vi "Normalized Axes.vi"(8 "axis in":T3, 11 "Device in":T1={"device ID"=refnum, "Device Name"="Logitech Extreme 3D", "axis info"={"X axis"=[], "Y axis"=[], "Z axis"=[], "X axis rotation"=[], "Y axis rotation"=[], "Z axis rotation"=[], "U axis"=[], "V axis"=[]}}) -> (0 "axis out":T2, 3 "Device out":T1={"device ID"=refnum, "Device Name"="Logitech Extreme 3D", "axis info"={"X axis"=[], "Y axis"=[], "Z axis"=[], "X axis rotation"=[], "Y axis rotation"=[], "Z axis rotation"=[], "U axis"=[], "V axis"=[]}})   [LabVIEW 2012]
doc: "This VI is used to normalize the newly reed axis info utilizing past minimums and maximums found during the calibration process. This ensures that the control input remains within the bounded range of 1 to -1.\nRuffin"
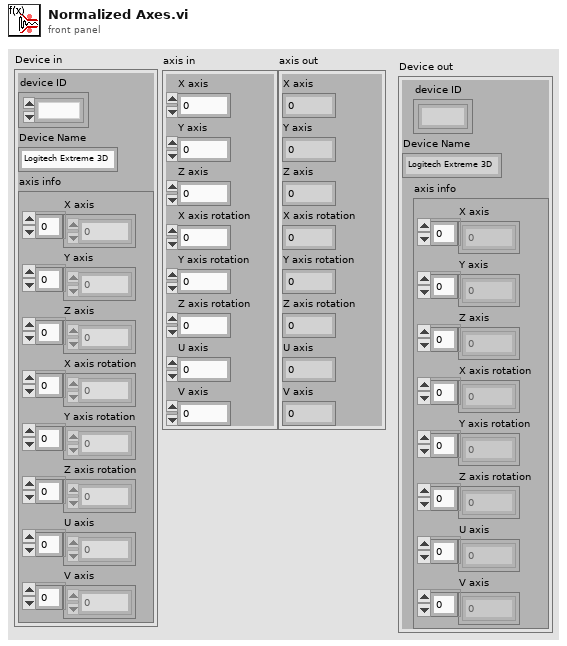
[diagram p1: front panel]
types:
  T1 = cluster{"device ID":refnum<k1>, "Device Name":string, "axis info":cluster{"X axis":dbl[], "Y axis":dbl[], "Z axis":dbl[], "X axis rotation":dbl[], "Y axis rotation":dbl[], "Z axis rotation":dbl[], "U axis":dbl[], "V axis":dbl[]}}
  T2 = cluster{"X axis":dbl, "Y axis":dbl, "Z axis":dbl, "X axis rotation":dbl, "Y axis rotation":dbl, "Z axis rotation":dbl, "U axis":dbl, "V axis":dbl}
  T3 = cluster{"X axis":i32, "Y axis":i32, "Z axis":i32, "X axis rotation":i32, "Y axis rotation":i32, "Z axis rotation":i32, "U axis":i32, "V axis":i32}
  T4 = cluster{"X axis":dbl[], "Y axis":dbl[], "Z axis":dbl[], "X axis rotation":dbl[], "Y axis rotation":dbl[], "Z axis rotation":dbl[], "U axis":dbl[], "V axis":dbl[]}
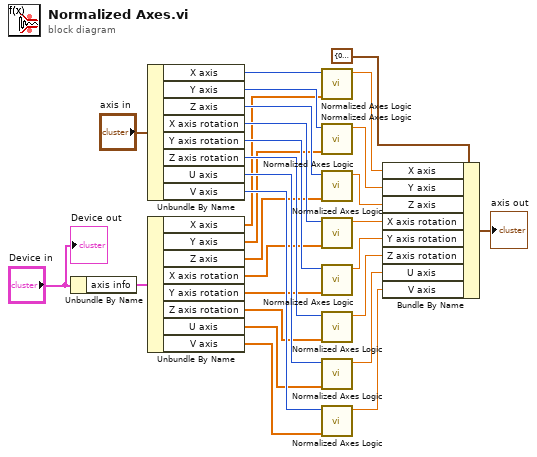
[diagram p0: block diagram]
diagram:
  n1 = Unbundle By Name("Device in") -> ("axis info"=w26:T4)
  n2 = Unbundle By Name("axis in") -> ("X axis"=w24:i32, "Y axis"=w22:i32, "Z axis"=w21:i32, "X axis rotation"=w20:i32, "Y axis rotation"=w19:i32, "Z axis rotation"=w18:i32, "U axis"=w17:i32, "V axis"=w16:i32)
  n3 = Unbundle By Name(w26) -> ("X axis"=w15:dbl[], "Y axis"=w14:dbl[], "Z axis"=w13:dbl[], "X axis rotation"=w12:dbl[], "Y axis rotation"=w11:dbl[], "Z axis rotation"=w10:dbl[], "U axis"=w9:dbl[], "V axis"=w8:dbl[])
  n4 = call "Normalized Axes Logic.vi"("axis"=w15, "axis in"=w24) -> ("axis out"=w23:dbl)  [unwired: 9 in]
  n5 = call "Normalized Axes Logic.vi"("axis"=w14, "axis in"=w22) -> ("axis out"=w7:dbl)  [unwired: 9 in]
  n6 = call "Normalized Axes Logic.vi"("axis"=w13, "axis in"=w21) -> ("axis out"=w6:dbl)  [unwired: 9 in]
  n7 = call "Normalized Axes Logic.vi"("axis"=w12, "axis in"=w20) -> ("axis out"=w5:dbl)  [unwired: 9 in]
  n8 = call "Normalized Axes Logic.vi"("axis"=w11, "axis in"=w19) -> ("axis out"=w4:dbl)  [unwired: 9 in]
  n9 = call "Normalized Axes Logic.vi"("axis"=w10, "axis in"=w18) -> ("axis out"=w3:dbl)  [unwired: 9 in]
  n10 = call "Normalized Axes Logic.vi"("axis"=w9, "axis in"=w17) -> ("axis out"=w2:dbl)  [unwired: 9 in]
  n11 = call "Normalized Axes Logic.vi"("axis"=w8, "axis in"=w16) -> ("axis out"=w1:dbl)  [unwired: 9 in]
  n12 = Bundle By Name(cluster=T2 {"X axis"=0.0, "Y axis"=0.0, "Z axis"=0.0, "X axis rotation"=0.0, "Y axis rotation"=0.0, "Z axis rotation"=0.0, "U axis"=0.0, "V axis"=0.0} ("axis info out"), "X axis"=w23, "Y axis"=w7, "Z axis"=w6, "X axis rotation"=w5, "Y axis rotation"=w4, "Z axis rotation"=w3, "U axis"=w2, "V axis"=w1) -> (→"axis out":T2)
  "Device out" <- "Device in"
